vi "DeInit.vi"(8 "error in (no error)":errorcluster, 11 "KeysightN9020B in":refnum<class "KeysightN9020B.lvclass">) -> (0 "error out":errorcluster, 3 "KeysightN9020B out":refnum<class "KeysightN9020B.lvclass">)   [LabVIEW 2023, in "KeysightN9020B.lvlib" / "KeysightN9020B.lvclass"]
uses:
  KeysightN9020B.lvclass
  C:/Program Files/National Instruments/LabVIEW 2023/vi.lib/ActorFramework/Actor/Actor.lvclass
  <vilib>/ActorFramework/Actor/Actor.lvclass/Actor.ctl
  KeysightN9020B.lvclass/KeysightN9020B.ctl
  Interfaces/InitDeinitInterface/InitDeinitComm Messages/DeInit Done Msg/DeInit Done Msg.lvclass/DeInit Done Msg.ctl
  <vilib>/ActorFramework/Message Enqueuer/Message Enqueuer.lvclass/Message Enqueuer.ctl
  <vilib>/ActorFramework/Message Enqueuer/Enqueue.vi
  Interfaces/InitDeinitInterface/InitDeinitComm Messages/DeInit Done Msg/DeInit Done Msg.lvclass
  C:/Program Files/National Instruments/LabVIEW 2023/vi.lib/ActorFramework/Message/Message.lvclass
  <vilib>/ActorFramework/Message Priority Queue/Priority Enqueue.vi
  <vilib>/ActorFramework/Actor/Actor.lvclass
  <instrlib>/Keysight XSAn/Keysight XSAn.lvlib
  C:/Users/DELL/Documents/LVDAQ/ConcreteClasses/ConcreteInstrumentClasses/KeysightN9020B/KeysightN9020B.lvclass
  C:/Users/DELL/Documents/LVDAQ/Interfaces/AbstractInstrumentClasses/SpectrumAnalyzer_LV/SpectrumAnalyzerInterface/SpectrumAnalyzer.lvclass
  C:/Users/DELL/Documents/LVDAQ/Interfaces/InitDeinitInterface/InitDeinit/InitDeinit.lvclass
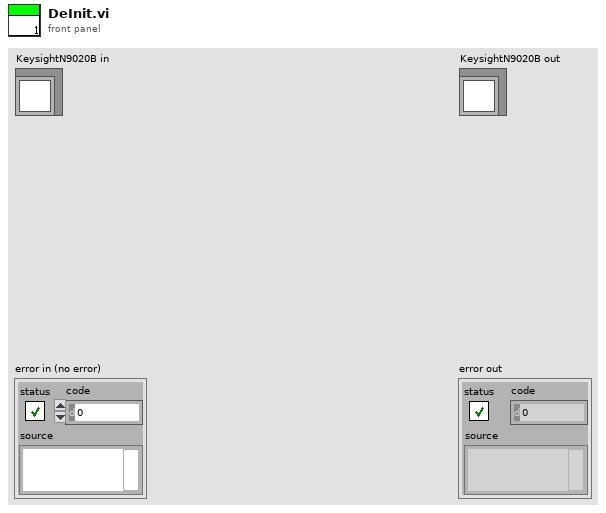
[diagram p1: front panel]
types:
  T1 = typedef "typedefs.lvlib/InstrumentData.ctl" = cluster{"Instr Error":errorcluster, "Address":cluster{"address type":enum16{"VISA", "Index"}, "Address":string, "instrument type":T2}, "CurrentState":cluster{"Initialized":bool, "Connected":bool, "Running":bool, "Error":bool}}
  T2 = typedef "typedefs.lvlib/instrumentType.ctl" = enum16{"Spectrum Analyzer", "Spectrometer", "Camera", "Stepper", "Piezo", "SLM"}
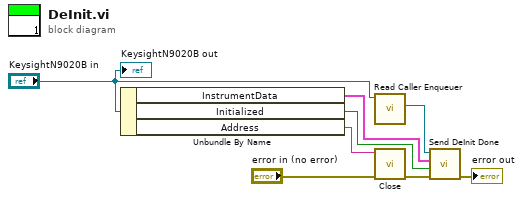
[diagram p0: block diagram]
diagram:
  n1 = Unbundle By Name("KeysightN9020B in") -> ("InstrumentData"=w6:T1, "Initialized"=w4:bool, "Address"=w3:string)
  n2 = call <vilib>:"Read Caller Enqueuer.vi"("Actor"="KeysightN9020B in") -> ("Caller Enqueuer"=w8:refnum<class "Message Enqueuer.lvclass">)  [unwired: 10 in]
  n3 = call <instrlib>:"Close.vi"("error in (no error)"="error in (no error)", "instrument handle"=w3) -> ("error out"=w1:errorcluster)  [unwired: 9 in]
  n4 = call "Send DeInit Done.vi"("error in (no error)"=w1, "Initialized"=w4, "InstrumentData"=w6, "Message Enqueuer"=w8) -> ("error out"=→"error out":errorcluster)  [unwired: 6 in, 1 out]
  "KeysightN9020B out" <- "KeysightN9020B in"
